vi "test Connect.vi"(8 "error in (no error)":errorcluster, 11 "TestCase in":refnum<class "SLSC Switch Messaging Tests.lvclass">) -> (0 "error out":errorcluster, 3 "TestCase out":refnum<class "SLSC Switch Messaging Tests.lvclass">)   [LabVIEW 2017, in "SLSC Switch Messaging Tests.lvclass"]
uses:
  SLSC Switch Messaging Tests.lvclass
  SLSC-Switch-Simulator/Includes/CDMessaging.lvlibp/Switch/Switch Connect Message/Switch Connect Message.lvclass
  C:/dev/CustomDevice/niveristand-slsc-switch-message-library/Includes/CDMessaging.lvlibp/Message/Abstract Message/Abstract Message.lvclass
  Support/Mock SLSC Switch Consumer.lvclass
  SLSC Switch Messaging Tests.lvclass/SLSC Switch Messaging Tests.ctl
  Support/Mock SLSC Switch Consumer.lvclass/Mock SLSC Switch Consumer.ctl
  Support/Read Connections.vi
  SLSC-Switch-Simulator/Includes/CDMessaging.lvlibp/Switch/Abstract Switch Consumer/Abstract Switch Consumer.lvclass
  C:/dev/CustomDevice/niveristand-slsc-switch-message-library/Includes/CDMessaging.lvlibp/Consumer/Abstract Consumer/Abstract Consumer.lvclass
  SLSC-Switch-Simulator/Includes/CDMessaging.lvlibp/Producer/Abstract Producer/Abstract Producer.lvclass
  <vilib>/addons/_JKI Toolkits/VI Tester/TestCase.llb/TestCase.lvclass
  SLSC-Switch-Simulator/Includes/CDMessaging.lvlibp/Consumer/Abstract Consumer/Abstract Consumer.lvclass
  C:/Program Files (x86)/National Instruments/LabVIEW 2017/vi.lib/addons/_JKI Toolkits/VI Tester/TestCase.llb/TestCase.lvclass
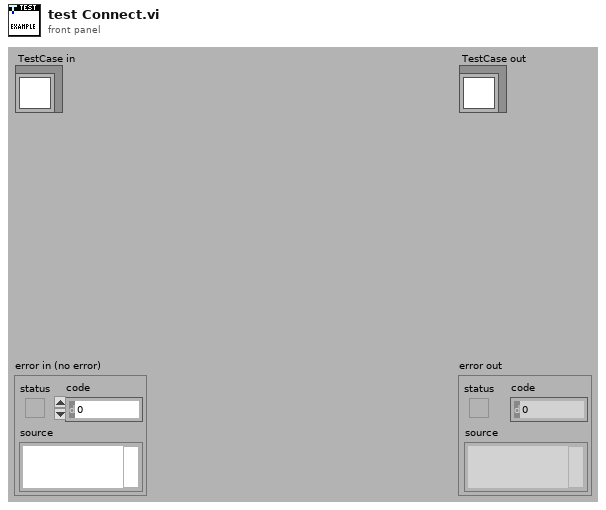
[diagram p1: front panel]
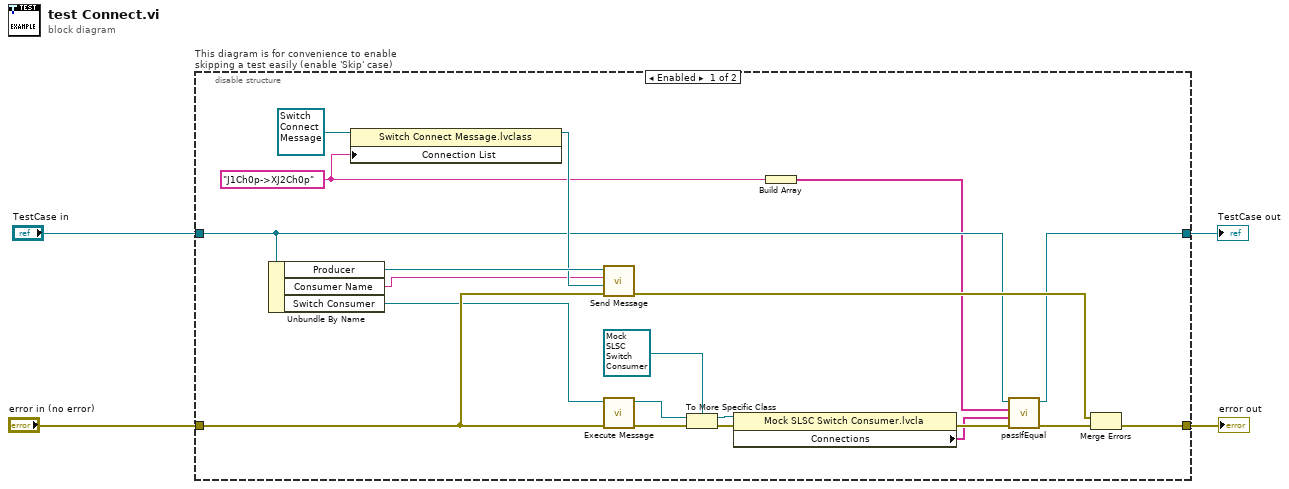
[diagram p0: block diagram]
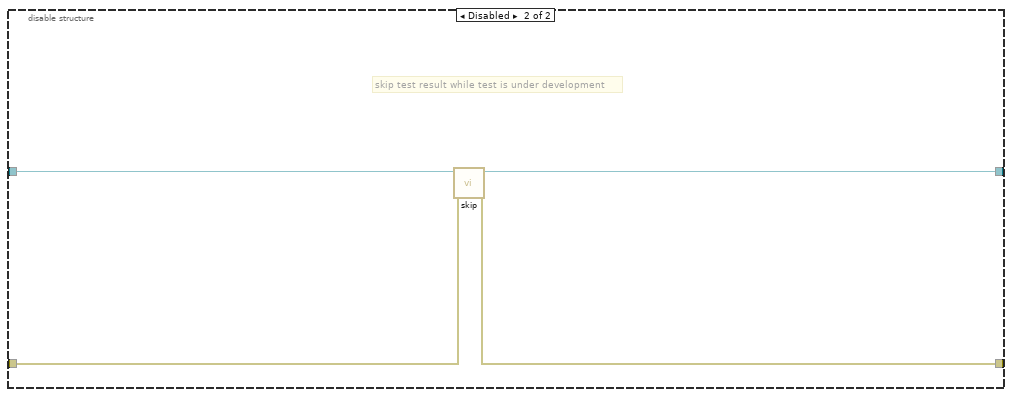
[diagram p2: hidden frame]
diagram:
  n1 = disable-structure "This diagram is for convenience to enable skipping a test easily (enable 'Skip' case)" shown="Enabled" {
    disable-tunnel: "TestCase in" -> [w8 w28]
    disable-tunnel: [w7 w26] -> w1
    disable-tunnel: [w17 w27] -> w3
    disable-tunnel: "error in (no error)" -> [w20 w25]
    frame Enabled {
      w10 = "J1Ch0p->XJ2Ch0p"
      n2 = Unbundle By Name(w8) -> ("Producer"=w23:refnum<class "Abstract Producer.lvclass">, "Consumer Name"=w21:string, "Switch Consumer"=w19:refnum<class "Abstract Switch Consumer.lvclass">)
      n3 = property class="Switch Connect Message.lvclass"(reference=refnum<class "Switch Connect Message.lvclass"> refnum ("CDMessaging.lvlibp:Switch Connect Message.lvclass"), "Connection List"=w10) -> (reference out=w22:refnum<class "Switch Connect Message.lvclass">)  [unwired: 1 in, 1 out]
      n4 = call-dynamic "Send Message.vi"("error in (no error)"=w20, "Message in"=w22, "Consumer in"=w21, "Abstract Producer in"=w23) -> ("error out"=w18:errorcluster)  [unwired: 4 in, 3 out]
      n5 = call "Execute Message.vi"("error in (no error)"=w20, "Abstract Consumer in"=w19) -> ("error out"=w16:errorcluster, "Abstract Consumer out"=w14:refnum<class "Abstract Consumer.lvclass">)  [unwired: 7 in, 1 out]
      n6 = To More Specific Class(target class=refnum<class "Mock SLSC Switch Consumer.lvclass"> refnum ("Mock SLSC Switch Consumer.lvclass"), reference=w14, error in=w16) -> (specific class reference=w11:refnum<class "Mock SLSC Switch Consumer.lvclass">, error out=w13:errorcluster)
      n7 = property class="Mock SLSC Switch Consumer.lvcla"(reference=w11, error in=w13) -> (error out=w12:errorcluster, "Connections"=w5:string[])  [unwired: 1 out]
      n8 = Build Array(w10) -> (w6:string[])
      n9 = call-dynamic "passIfEqual.vi"("error in (no error)"=w12, "y"=w5, "x"=w6, "TestCase in"=w8) -> ("error out"=w9:errorcluster, "TestCase out"=w7:refnum<class "SLSC Switch Messaging Tests.lvclass">)  [unwired: 6 in]
      n10 = Merge Errors(w18, w9) -> (w17:errorcluster)
    }
    frame Disabled {
      # "skip test result while test is under development"
      n11 = call <vilib>:"skip.vi"("error in (no error)"=w25, "TestCase in"=w28) -> ("error out"=w27:errorcluster, "TestCase out"=w26:refnum<class "SLSC Switch Messaging Tests.lvclass">)  [unwired: 8 in]
    }
  }
  "error out" <- w3
  "TestCase out" <- w1
